vi "GetCameraChanBySerialNumber.vi"(10 "camera serial number":string, 11 "channels":T1[](array[typedef])) -> (1 "found":bool, 2 "channel (camera)":T1, 3 "channels out":T1[](array[typedef]))   [LabVIEW 2017, in "DeviceModelHelpers.lvlib"]
uses:
  <vilib>/addons/InsightCM/Utilities/DeviceModelHelpers/DeviceModelHelpers.lvlib
  <vilib>/addons/InsightCM/MessageBus/Base/controls/R2_Channel.ctl
  <vilib>/addons/InsightCM/MessageBus/Base/controls/KeyValuePair.ctl
  <vilib>/addons/InsightCM/MessageBus/Base/controls/Metric.ctl
  <vilib>/addons/InsightCM/Utilities/PropertyHelpers/PropertyHelpers.lvlib
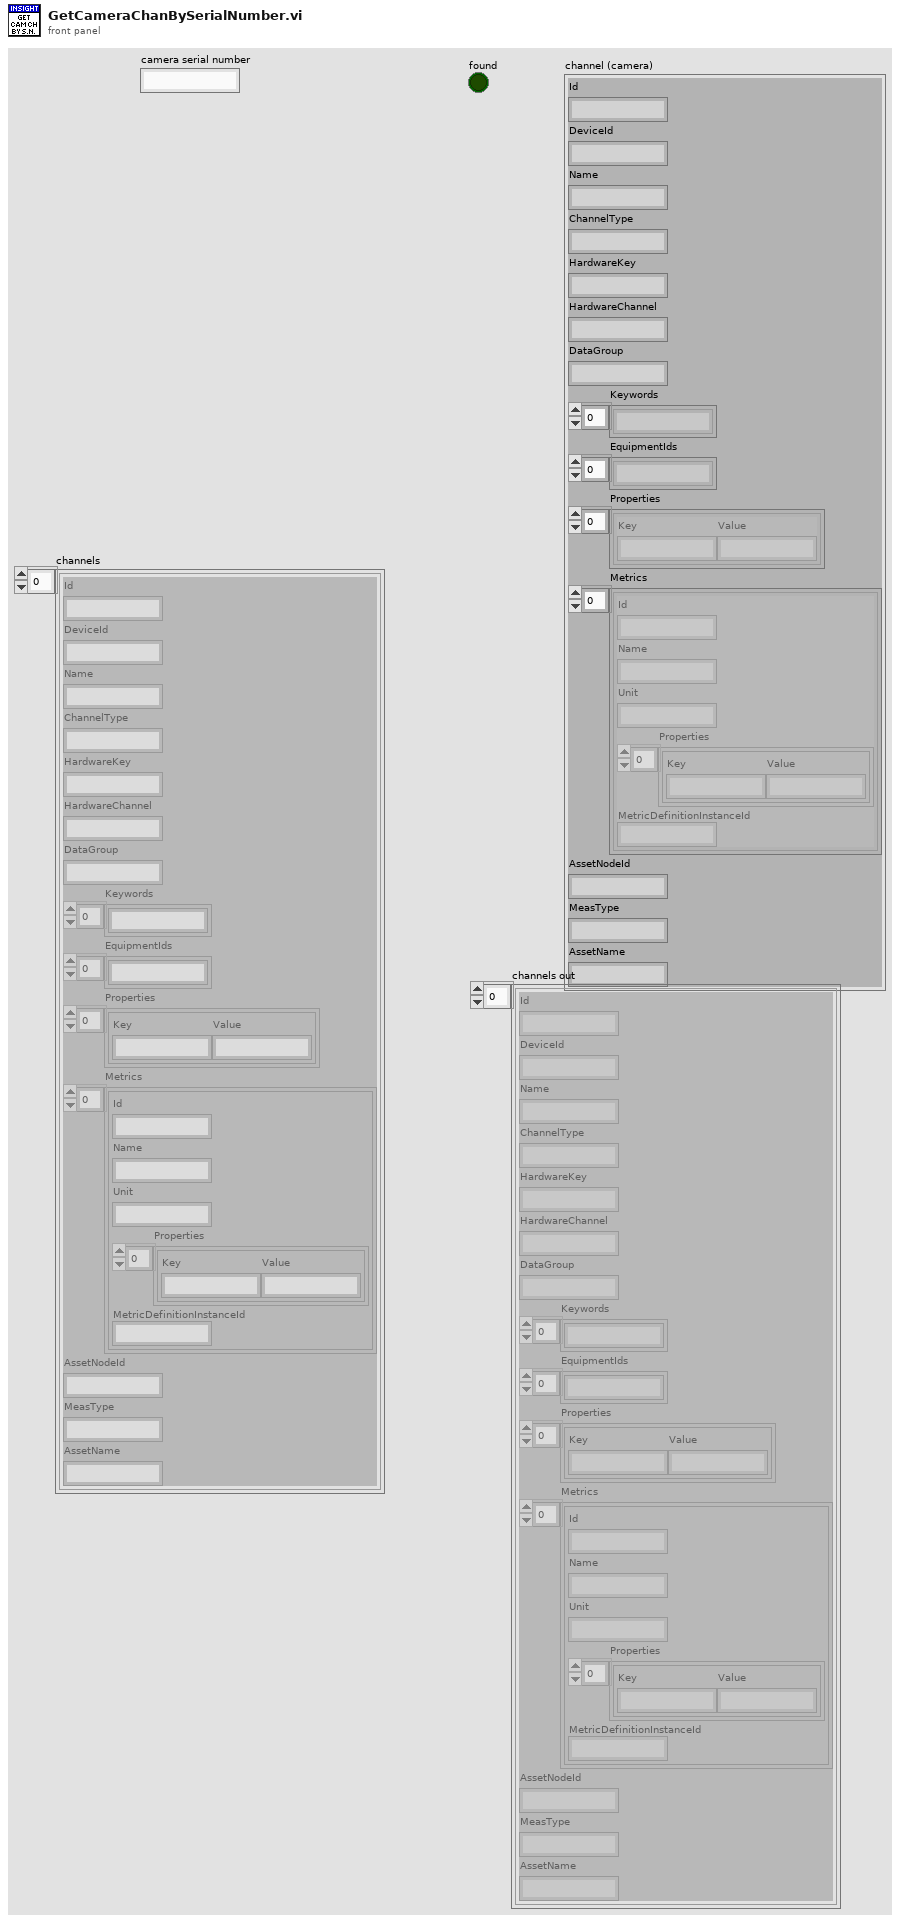
[diagram p1: front panel]
types:
  T1 = typedef "R2_Channel.ctl" = cluster{"Id":string, "DeviceId":string, "Name":string, "ChannelType":string, "HardwareKey":string, "HardwareChannel":string, "DataGroup":string, "Keywords":string[], "EquipmentIds":string[], "Properties":T2[], "Metrics":T3[], "AssetNodeId":string, "MeasType":string, "AssetName":string}
  T2 = typedef "KeyValuePair.ctl" = cluster{"Key":string, "Value":string}
  T3 = typedef "Metric.ctl" = cluster{"Id":string, "Name":string, "Unit":string, "Properties":T2[], "MetricDefinitionInstanceId":string}
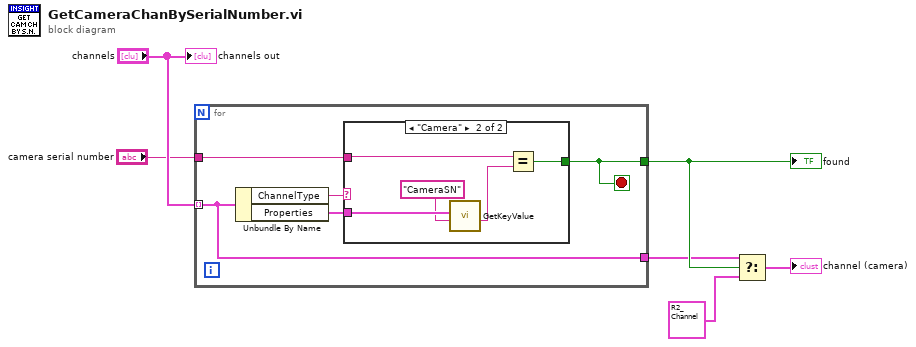
[diagram p0: block diagram]
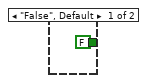
[diagram p2: hidden frame]
diagram:
  n1 = for {
    tunnel: "channels" -> [w8] mode=indexing
    tunnel: "camera serial number" -> [w9]
    tunnel: [w8] -> w3
    tunnel: [w7] -> w4
    stop <- w7 stop-if-true
    n2 = Unbundle By Name(w8) -> ("ChannelType"=w11:string, "Properties"=w10:T2[])
    n3 = case shown="\"Camera\"" w11 {
      tunnel: w10 -> [_ w17]
      tunnel: w9 -> [_ w15]
      tunnel: [FALSE w13] -> w7
      frame "False", Default {
      }
      frame "Camera" {
        n4 = call <vilib>:"GetKeyValue.vi"("key"="CameraSN", "key value pairs"=w17) -> ("value"=w14:string)  [unwired: 7 in, 2 out]
        n5 = Equal?(x=w15, y=w14) -> (x = y?=w13:bool)
      }
    }
  }
  "found" <- w4
  n6 = Select(t=w3, s=w4, f=T1 {"Id"="", "DeviceId"="", "Name"="", "ChannelType"="", "HardwareKey"="", "HardwareChannel"="", "DataGroup"="", "Keywords"=[], "EquipmentIds"=[], "Properties"=[], "Metrics"=[], "AssetNodeId"="", "MeasType"="", "AssetName"=""}) -> (s? t:f=→"channel (camera)":T1)
  "channels out" <- "channels"
